vi "固定站氨氮测量流程.vi"(11 "控制命令":T1(ring)) -> ()   [LabVIEW 2016, in "斯坦道氨氮.lvlib"]
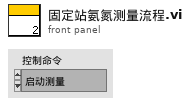
[diagram p1: front panel]
types:
  T1 = enum16{"启动测量", "标样核查", "零点核查", "跨度核查", "空白测试", "平行样测试", "加标回收", "空白校准", "标样校准", "初始化（清洗）", "停止测试", "仪器重启", "校时", "模式设置", "测量间隔设置"}
  T2 = cluster{"仪器":enum16{"", "氨氮", "总磷", "总氮", "CODMn", "CODCr"}, "启动命令":enum16{"启动水样流程", "启动加标流程", "排液", "停止", "柱塞泵启动"}}
  T3 = cluster{"时间标识":timestamp, "设备":string, "日志信息":string, "流程参数":string}
  T4 = cluster{"站号":u16, "量程切换":enum32{"H", "L", "AUTO"}, "控制命令":enum16{"启动测量", "标样核查", "零点核查", "跨度核查", "空白测试", "平行样测试", "加标回收", "空白校准", "标样校准", "初始化（清洗）", "停止测试", "仪器重启", "校时", "模式设置", "测量间隔设置"}, "模式设置":enum16{"待机", "连续模式", "周期模式", "定点模式", "受控模式", "手动模式"}, "测量间隔":u16}
  T5 = cluster{"系统时间":timestamp, "工作状态":enum16{"空闲", "水样测试", "标样核查", "零点核查", "跨度核查", "空白测试", "平行样测试", "加标回收", "空白校准", "标样校准", "初始化（清洗）"}, "测量模式":enum16{"待机", "连续模式", "周期模式", "定点模式", "受控模式", "手动模式"}, "告警代码":u16, "故障代码":u16, "日志代码":u16, "软件版本":u16, "F0":sgl, "F1":sgl, "F2":sgl, "F3":sgl, "T":sgl, "H":sgl, "id":u16, "flowid":u16, "量程":u16, "总磷控温温度1":sgl, "营养盐控温温度2":sgl, "ADC":sgl}
  T6 = cluster{"水样测试量程模式":enum16{"H", "L", "AUTO"}, "空白核查量程模式":enum16{"H", "L", "AUTO"}, "跨度核查量程模式":enum16{"H", "L", "AUTO"}}
  T7 = enum16{"空闲", "水样测试", "标样核查", "零点核查", "跨度核查", "空白测试", "平行样测试", "加标回收", "空白校准", "标样校准", "初始化（清洗）"}
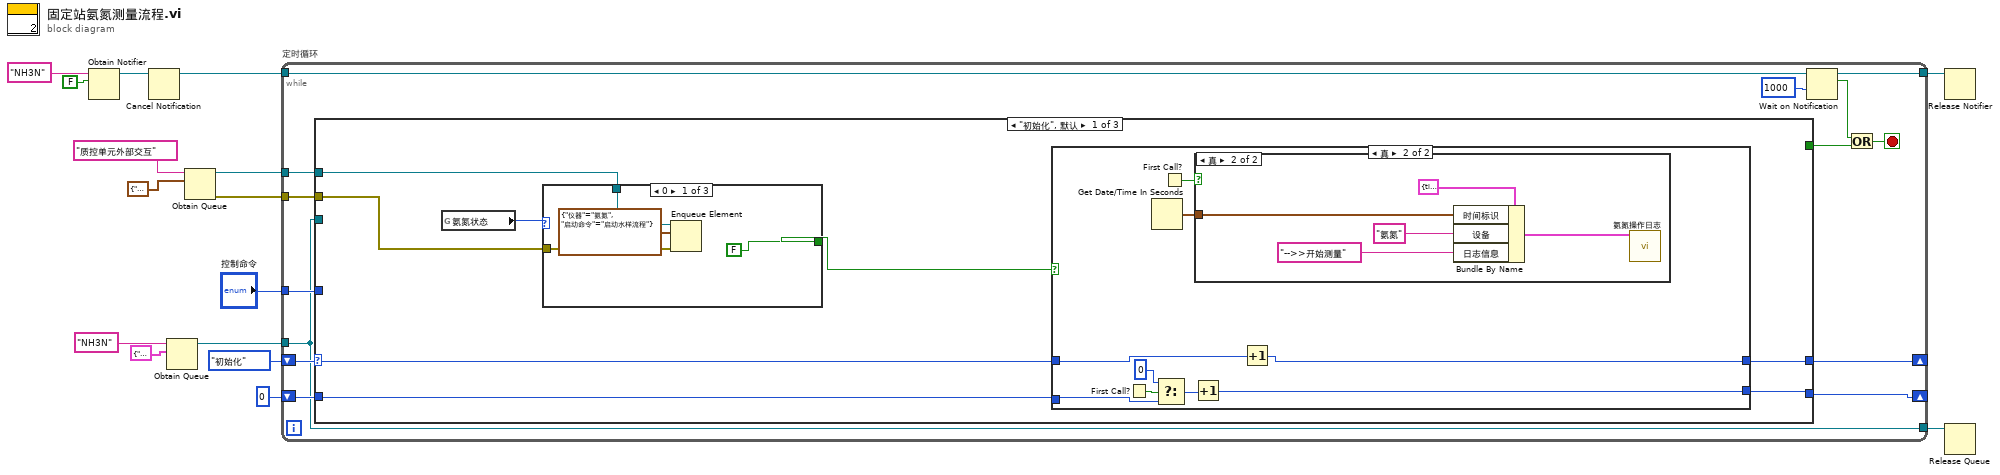
[diagram p0: block diagram]
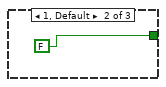
[diagram p4: hidden frame]
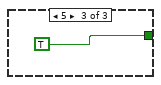
[diagram p5: hidden frame]
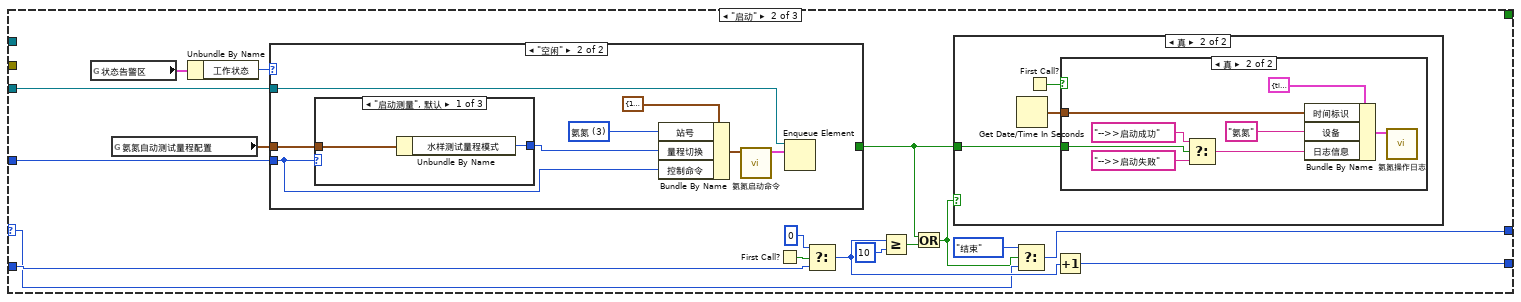
[diagram p6: hidden frame]
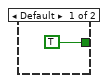
[diagram p9: hidden frame]
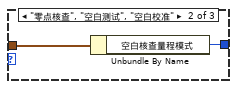
[diagram p10: hidden frame]
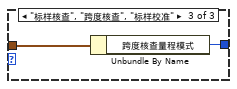
[diagram p11: hidden frame]
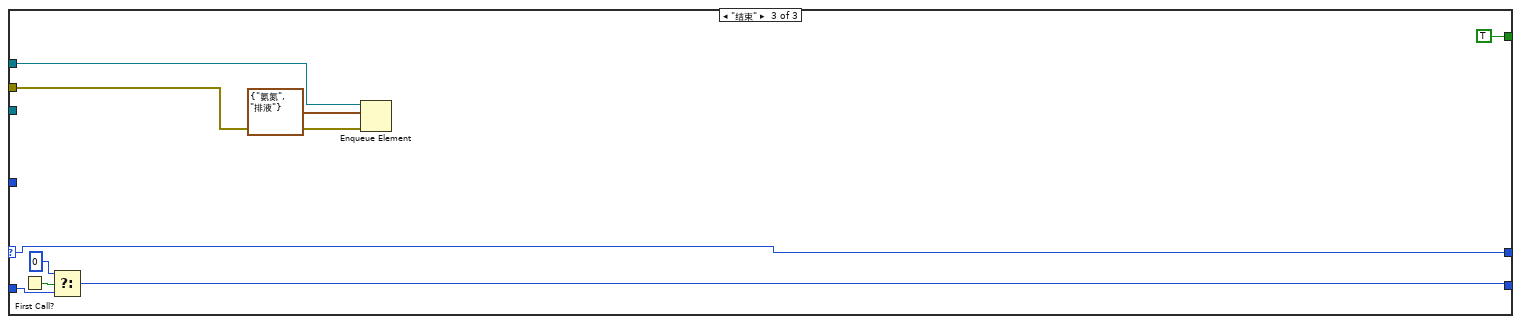
[diagram p12: hidden frame]
diagram:
  n1 = Obtain Notifier(name (unnamed)="NH3N" ("名称（未命名）"), notification data type=FALSE) -> (notifier out=w11:refnum<notifier>)  [unwired: 2 in, 2 out]
  n2 = Cancel Notification(0:w11) -> (8:w10:refnum<notifier>)  [unwired: 1 in, 2 out]
  n3 = Obtain Queue(name (unnamed)="NH3N" ("名称（未命名）"), element data type=cluster{"命令":string, "data":variant} {"命令"="", "data"=variant}) -> (queue out=w14:refnum<queue>)  [unwired: 3 in, 2 out]
  n4 = Obtain Queue(name (unnamed)="质控单元外部交互" ("名称（未命名）"), element data type=T2 {"仪器"=enum."氨氮", "启动命令"=enum."启动水样流程"} ("元素")) -> (queue out=w2:refnum<queue>, error out=w1:errorcluster)  [unwired: 3 in, 1 out]
  n5 = while "定时循环" {
    tunnel: w14 -> [w19]
    tunnel: w10 -> [w30]
    tunnel: "控制命令" -> [w25]
    shift-right: [w24] -> _
    shift-left: enum16{"初始化", "启动", "结束"}."初始化" -> [w26]
    shift-right: [w22] -> _
    shift-left: 0 -> [w23]
    tunnel: [w20] -> w6
    tunnel: [w19] -> w7
    tunnel: w2 -> [w18]
    tunnel: w1 -> [w17]
    stop <- w27 stop-if-true
    n6 = case shown="\"初始化\", 默认" w26 {
      selector: w26 -> [w38 w66 w112]
      tunnel: w25 -> [_ w77 _]
      tunnel: w19 -> [_ w76 _]
      tunnel: [w37 w67 w112] -> w24
      tunnel: w23 -> [w36 w71 w109]
      tunnel: [w35 w70 w108] -> w22
      tunnel: [_ _ TRUE] -> w21
      tunnel: w18 -> [w32 _ w105]
      tunnel: w17 -> [w31 _ w104]
      frame "初始化", Default {
        n7 = global read "VAR氨氮全局变量.vi" "氨氮状态"() -> (w33:u16)
        n8 = case shown="0" w33 {
          tunnel: [FALSE ("s") FALSE ("s") TRUE ("s")] -> w34
          tunnel: w32 -> [w57 _ _]
          tunnel: w31 -> [w56 _ _]
          frame 0 {
            n9 = Enqueue Element(queue=w57, element=T2 {"仪器"=enum."氨氮", "启动命令"=enum."启动水样流程"} ("元素"), error in (no error)=w56) -> ()  [unwired: 1 in, 3 out]
          }
          frame 1, Default {
          }
          frame 5 {
          }
        }
        n10 = case shown="真" w34 {
          tunnel: w38 -> [w40 w47]
          tunnel: [w40 w46] -> w37
          tunnel: w36 -> [w39 w44]
          tunnel: [w39 w41] -> w35
          frame False {
          }
          frame True {
            n11 = First Call?() -> (First Call?: T/F=w45:bool)
            n12 = Get Date/Time In Seconds() -> (seconds since 1Jan1904=w49:timestamp)
            n13 = Select(t=0, s=w45, f=w44) -> (s? t:f=w42:i32)
            n14 = First Call?() -> (First Call?: T/F=w48:bool)
            n15 = Increment(x=w42) -> (x+1=w41:i32)
            n16 = case shown="真" w48 {
              tunnel: w49 -> [_ w53]
              frame False {
              }
              frame True {
                n17 = Bundle By Name(cluster=T3 {"时间标识"=timestamp(0 s since 1904-01-01), "设备"="", "日志信息"="", "流程参数"=""} ("data in"), "时间标识"=w53, "设备"="氨氮", "日志信息"="-->>开始测量") -> (w54:T3)
                n18 = call "氨氮操作日志.vi"("data in"=w54) -> ()  [unwired: 11 in]
              }
            }
            n19 = Increment(x=w47) -> (x+1=w46:enum16{"初始化", "启动", "结束"})
          }
        }
      }
      frame "启动" {
        n20 = global read "VAR氨氮全局变量.vi" "状态告警区"() -> (w75:T5)
        n21 = global read "氨氮断电保存全局变量.vi" "氨氮自动测试量程配置"() -> (w61:T6)
        n22 = Unbundle By Name(w75) -> ("工作状态"=w74:T7)
        n23 = case shown="\"空闲\"" w74 {
          tunnel: w61 -> [_ w95]
          tunnel: w77 -> [_ w90]
          tunnel: w76 -> [_ w94]
          tunnel: [TRUE _] -> w62
          frame Default {
          }
          frame "空闲" {
            w93 = u16 3 items=["总磷"=1, "总氮"=2, "氨氮"=3] ("站号")
            n24 = case shown="\"启动测量\", 默认" w90 {
              tunnel: w95 -> [w99 w101 w103]
              tunnel: [w98 w100 w102] -> w97
              frame "启动测量", Default {
                n25 = Unbundle By Name(w99) -> ("水样测试量程模式"=w98:enum16{"H", "L", "AUTO"})
              }
              frame "零点核查", "空白测试", "空白校准" {
                n26 = Unbundle By Name(w101) -> ("空白核查量程模式"=w100:enum16{"H", "L", "AUTO"})
              }
              frame "标样核查", "跨度核查", "标样校准" {
                n27 = Unbundle By Name(w103) -> ("跨度核查量程模式"=w102:enum16{"H", "L", "AUTO"})
              }
            }
            n28 = Bundle By Name(cluster=T4 {"站号"=1, "量程切换"=enum."AUTO", "控制命令"=enum."启动测量", "模式设置"=enum."待机", "测量间隔"=0} ("参数"), "站号"=w93, "量程切换"=w97, "控制命令"=w90) -> (w91:T4)
            n29 = call "氨氮启动命令.vi"("参数"=w91) -> ("启动命令"=w96:cluster{"命令":string, "data":variant})  [unwired: 10 in]
            n30 = Enqueue Element(queue=w94, element=w96) -> ()  [unwired: 2 in, 3 out]
          }
        }
        n31 = First Call?() -> (First Call?: T/F=w73:bool)
        n32 = Select(t=0, s=w73, f=w71) -> (s? t:f=w69:i32)
        n33 = Greater Or Equal?(x=w69, y=10) -> (x >= y?=w65:bool)
        n34 = Or(x=w62, y=w65) -> (x .or. y?=w63:bool)
        n35 = case shown="真" w63 {
          tunnel: w62 -> [_ w78]
          frame False {
          }
          frame True {
            n36 = Get Date/Time In Seconds() -> (seconds since 1Jan1904=w79:timestamp)
            n37 = First Call?() -> (First Call?: T/F=w80:bool)
            n38 = case shown="真" w80 {
              tunnel: w79 -> [_ w87]
              tunnel: w78 -> [_ w84]
              frame False {
              }
              frame True {
                n39 = Select(t="-->>启动成功" ("日志信息"), s=w84, f="-->>启动失败" ("日志信息")) -> (s? t:f=w81:string)
                n40 = Bundle By Name(cluster=T3 {"时间标识"=timestamp(0 s since 1904-01-01), "设备"="", "日志信息"="", "流程参数"=""} ("data in"), "时间标识"=w87, "设备"="氨氮", "日志信息"=w81) -> (w88:T3)
                n41 = call "氨氮操作日志.vi"("data in"=w88) -> ()  [unwired: 11 in]
              }
            }
          }
        }
        n42 = Select(t=enum16{"初始化", "启动", "结束"}."结束", s=w63, f=w66) -> (s? t:f=w67:enum16{"初始化", "启动", "结束"})
        n43 = Increment(x=w69) -> (x+1=w70:i32)
      }
      frame "结束" {
        n44 = First Call?() -> (First Call?: T/F=w111:bool)
        n45 = Select(t=0, s=w111, f=w109) -> (s? t:f=w108:i32)
        n46 = Enqueue Element(queue=w105, element=T2 {"仪器"=enum."氨氮", "启动命令"=enum."排液"} ("元素"), error in (no error)=w104) -> ()  [unwired: 1 in, 3 out]
      }
    }
    n47 = Wait on Notification(notifier=w30, timeout in ms (-1)=1000 ("超时毫秒(-1)")) -> (notifier out=w20:refnum<notifier>, notification=w28:bool)  [unwired: 2 in, 2 out]
    n48 = Or(x=w28, y=w21) -> (x .or. y?=w27:bool)
  }
  n49 = Release Notifier(notifier=w6) -> ()  [unwired: 2 in, 3 out]
  n50 = Release Queue(queue=w7) -> ()  [unwired: 2 in, 3 out]
